vi "GTcode_v6_simulISS_MAP.vi"() -> ()   [LabVIEW 2016]
uses:
  <vilib>/Utility/config.llb/Write Key (String).vi
  <vilib>/Utility/config.llb/Write Key (U32).vi
  <vilib>/Utility/config.llb/Write Key (Double).vi
  <vilib>/Utility/config.llb/Write Key (I32).vi
  <vilib>/Utility/config.llb/Read Key (U32).vi
  <vilib>/Utility/config.llb/Read Key (I32).vi
  flex05-4chPascal.dll
  <vilib>/Utility/config.llb/NI_LVConfig.lvlib
  flex05oem8chauto100nsPASCAL_win7.dll
  <vilib>/Analysis/NI_AALBase.lvlib
panel:
  in  "Tab Control":T1(tab)=enum."Real Time Fitting Parameters"
  out "COV":dbl
  out "mean":dbl format="%0.2f"
  in  "Fixed Time":bool
  in  "Detector Used":T2(ring)=enum."Det 2"
  in  "Real Time Fitting?":bool
  out "g2":cluster{"Delay Time":sgl[], sgl[]}[](graph) caption="Normalized Correlation Function"
  out "Tau":cluster{"tmp":dbl, dbl}(graph) caption="Relative Changes of Flow"
  in  "QUIT":bool
  in  "Clear plots":bool
  in  "Baseline":bool
  in  "MARK\nMark":bool
  in  "Stop":bool
  in  "Sequence Scan":bool
  out "Mark #":u32
  out "Trial #":u32
  out "Frame #":u32
  out "Det 8":sgl format="%.3f"
  out "Det 7":sgl format="%.3f"
  out "Det 6":sgl format="%.3f"
  out "Det 5":sgl format="%.3f"
  out "Det 4":sgl format="%.3f"
  out "Det 3":sgl format="%.3f"
  out "Det 2":sgl format="%.3f"
  out "Det 1":sgl format="%.3f"
  out "Computer Time":string="2010-1-12 23:16:10"
  in  "D1":bool
  in  "D2":bool
  in  "D3":bool
  in  "D4":bool
  in  "D5":bool
  in  "D6":bool
  in  "D7":bool
  in  "D8":bool
  out "Tau 2":T3(graph)={1.6593152555505744e-08, 3.9427894777554196e-08, 4.065716407938411e-08, 1.5135790977358522e-08, 2.4870420100428357e-08, 7.094765128107397e-08, 0.0, 4.1348620928852906e-07, 1.5886917674344795e-08, 4.0280526032721455e-08, -1.0, -1.0} caption="Blood Flow Index (cm2/s)"
  in  "Fixed # of Frames":u32=5
  out "Status":string="Quit"
  in  "Optical Switch OPEN":bool
  in  "Delay between frames(ms)":u32=500
  out "Time Left (ms)":sgl format="%.3f"
  in  "Integration Time (ms)":sgl=1000.0 min=1 max=13000 step=1
  in  "File Name:":string="test0"
  in  "Data Save Directory:":path=path "C:/data"
  in  "ISS Lasers ON":bool
  in  "Test":bool
  in  "Lines":tag="Dev1/port1/line0:1, Dev1/port1/line3:7"
  in  "Delaytime(ms)":u32=200
  in  "Initialize Correlator":bool
  in  "Detector Select":enum32{"4 Detectors", "8 Detectors"}(radio)=enum."8 Detectors"
  in  "Update Time (ms)\nDO NOT CHANGE!":u32=105 min=1 max=999 step=1
  in  "Laser Input Name":refnum<visa-resource-name>="COM7"
  out "Flow in each detector":dbl[](array[numeric])=[-1.0, -1.0, -1.0, -1.0, -1.0, -1.0, -1.0, -1.0, -1.0, -1.0, -1.0, -1.0]
  in  "Visible Averages":bool[](array[boolean])=[FALSE, FALSE, FALSE, FALSE]
  in  "Avg":bool[][](array[boolean])=[[FALSE, FALSE, FALSE, FALSE, FALSE, FALSE, FALSE, FALSE], [FALSE, FALSE, FALSE, FALSE, FALSE, FALSE, FALSE, FALSE], [FALSE, FALSE, FALSE, FALSE, FALSE, FALSE, FALSE, FALSE], [FALSE, FALSE, FALSE, FALSE, FALSE, FALSE, FALSE, FALSE]]
  in  "rho":dbl[](array[numeric])=[2.5, 2.5, 2.5, 2.5, 2.5, 2.5, 2.5, 2.5, -1.0, -1.0, -1.0, -1.0]
  in  "Other Settings":u32[](array[numeric])=[1, 120, 0, 1] caption="Flow in each detector"
  in  "Initial Guess":dbl[](array[numeric])=[1e-08, 0.5, 0.05, 10.0] caption="Flow in each detector"
  in  "Number Samples":dbl=50.0
  out "NIBP Data (*scaled by 98 to convert from V to mmHg)":dynamicdata(graph)
  in  "Record MAP data?":bool=TRUE
  in  "Sampling Rate (Hz)":dbl=100.0
  in  "ExternalADC":tag="Dev2"
  out "4CH?":bool
  out "Detector#":u32=1
  out "Source#":u32=1
  # "kHz"
  # "kHz"
  # "Don't Change these Parameters unless you know clearly what you are doing"
  # "ISS Triggers Setup"
  # "Channel Parameters"
  # "Step1"
  # "Line"
  # "0"
  # "1"
  # "3"
  # "4"
  # "5"
  # "6"
  # "7"
  # "*The number of lines in the list must\nmatch the number of elements in\nthe array."
  # "Step2"
  # "Line"
  # "0"
  # "1"
  # "3"
  # "4"
  # "5"
  # "6"
  # "7"
  # "Step3"
  # "Line"
  # "0"
  # "1"
  # "3"
  # "4"
  # "5"
  # "6"
  # "7"
  # "Line    Signal\n\n0           ISS Trigger (0: OFF, 1: ON)\n1           Flow Laser 1 ON/OFF (0:OFF, 1:ON)\n2           ISS Data Acquisition (0: DONE, 1: NO)\n3           ISS Laser ON/OFF (0: ON, 1: OFF)\n4           Trigger for Marks  (0: OFF, 1: ON)\n5           Flow Laser 2 ON/OFF (0:OFF, 1:ON)\n6           Reserved\n7           Reserved"
  # "Wait ISS Data Acuisition DONE Signal"
  # "Step4"
  # "Step5"
  # "Line"
  # "0"
  # "1"
  # "3"
  # "4"
  # "5"
  # "6"
  # "7"
  # "Flow Lasers Setup"
  # "FROM FRONT PANEL"
  # "Line"
  # "0"
  # "1"
  # "3"
  # "4"
  # "5"
  # "6"
  # "7"
  # "Line"
  # "0"
  # "1"
  # "3"
  # "4"
  # "5"
  # "6"
  # "7"
  # "Det 1"
  # "Det 2"
  # "Det 3"
  # "Det 4"
  # "Det 5"
  # "Det 6"
  # "Det 7"
  # "Det 8"
  # "Avg 1"
  # "Avg 2"
  # "Avg 3"
  # "Avg 4"
  # "Db"
  # "Beta"
  # "Mua"
  # "MuS'"
  # "1"
  # "2"
  # "3"
  # "4"
  # "5"
  # "6"
  # "7"
  # "8"
  # "Avg 1"
  # "Starting Pt"
  # "End Pt"
  # "Approximate"
  # "Variables"
  # "Avg 2"
  # "Avg 3"
  # "Avg 4"
  # "Source Detector  Separations"
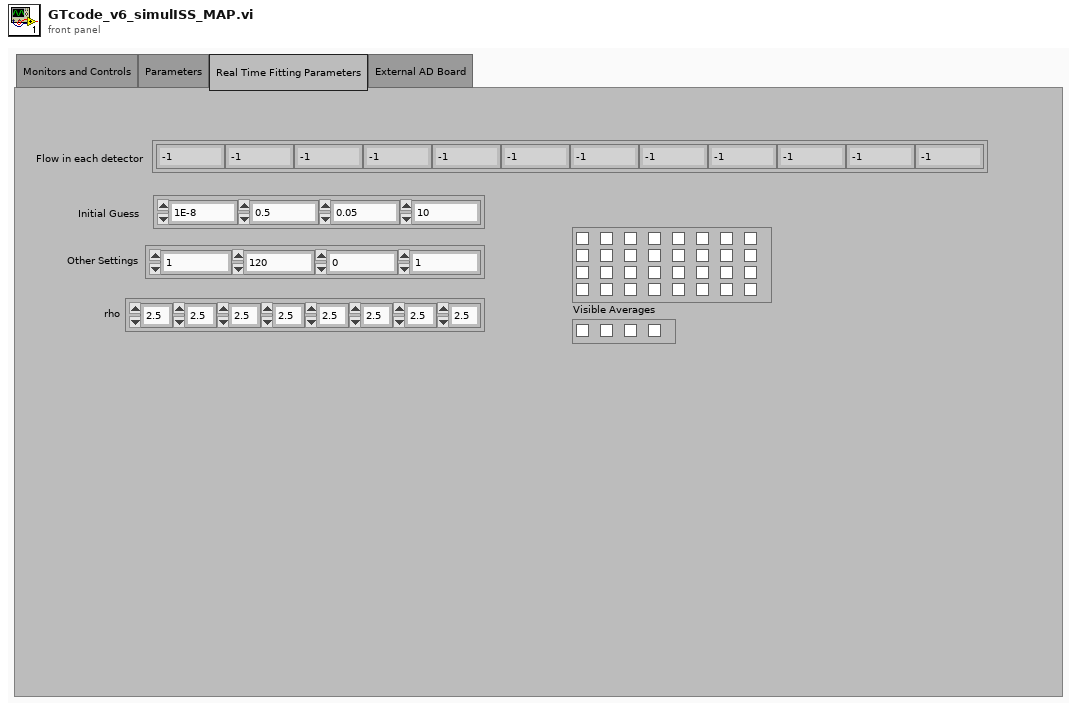
[diagram p1: front panel]
types:
  T1 = enum32{"Monitors and Controls", "Parameters", "Real Time Fitting Parameters", "External AD Board"}
  T2 = enum16{"Det 1", "Det 2", "Det 3", "Det 4", "Det 5", "Det 6", "Det 7", "Det 8"}
  T3 = cluster{dbl, dbl, dbl, dbl, dbl, dbl, dbl, dbl, dbl, dbl, dbl, dbl}
  T4 = enum8{"Enabled", "Disabled", "Disabled and Grayed Out"}
  T5 = cluster{dbl, dbl, dbl, dbl, dbl, dbl, dbl, dbl, dbl, dbl, dbl, dbl}[]
  T6 = typedef "NI_LVConfig.lvlib/Config Data RefNum.ctl" = refnum<k1>
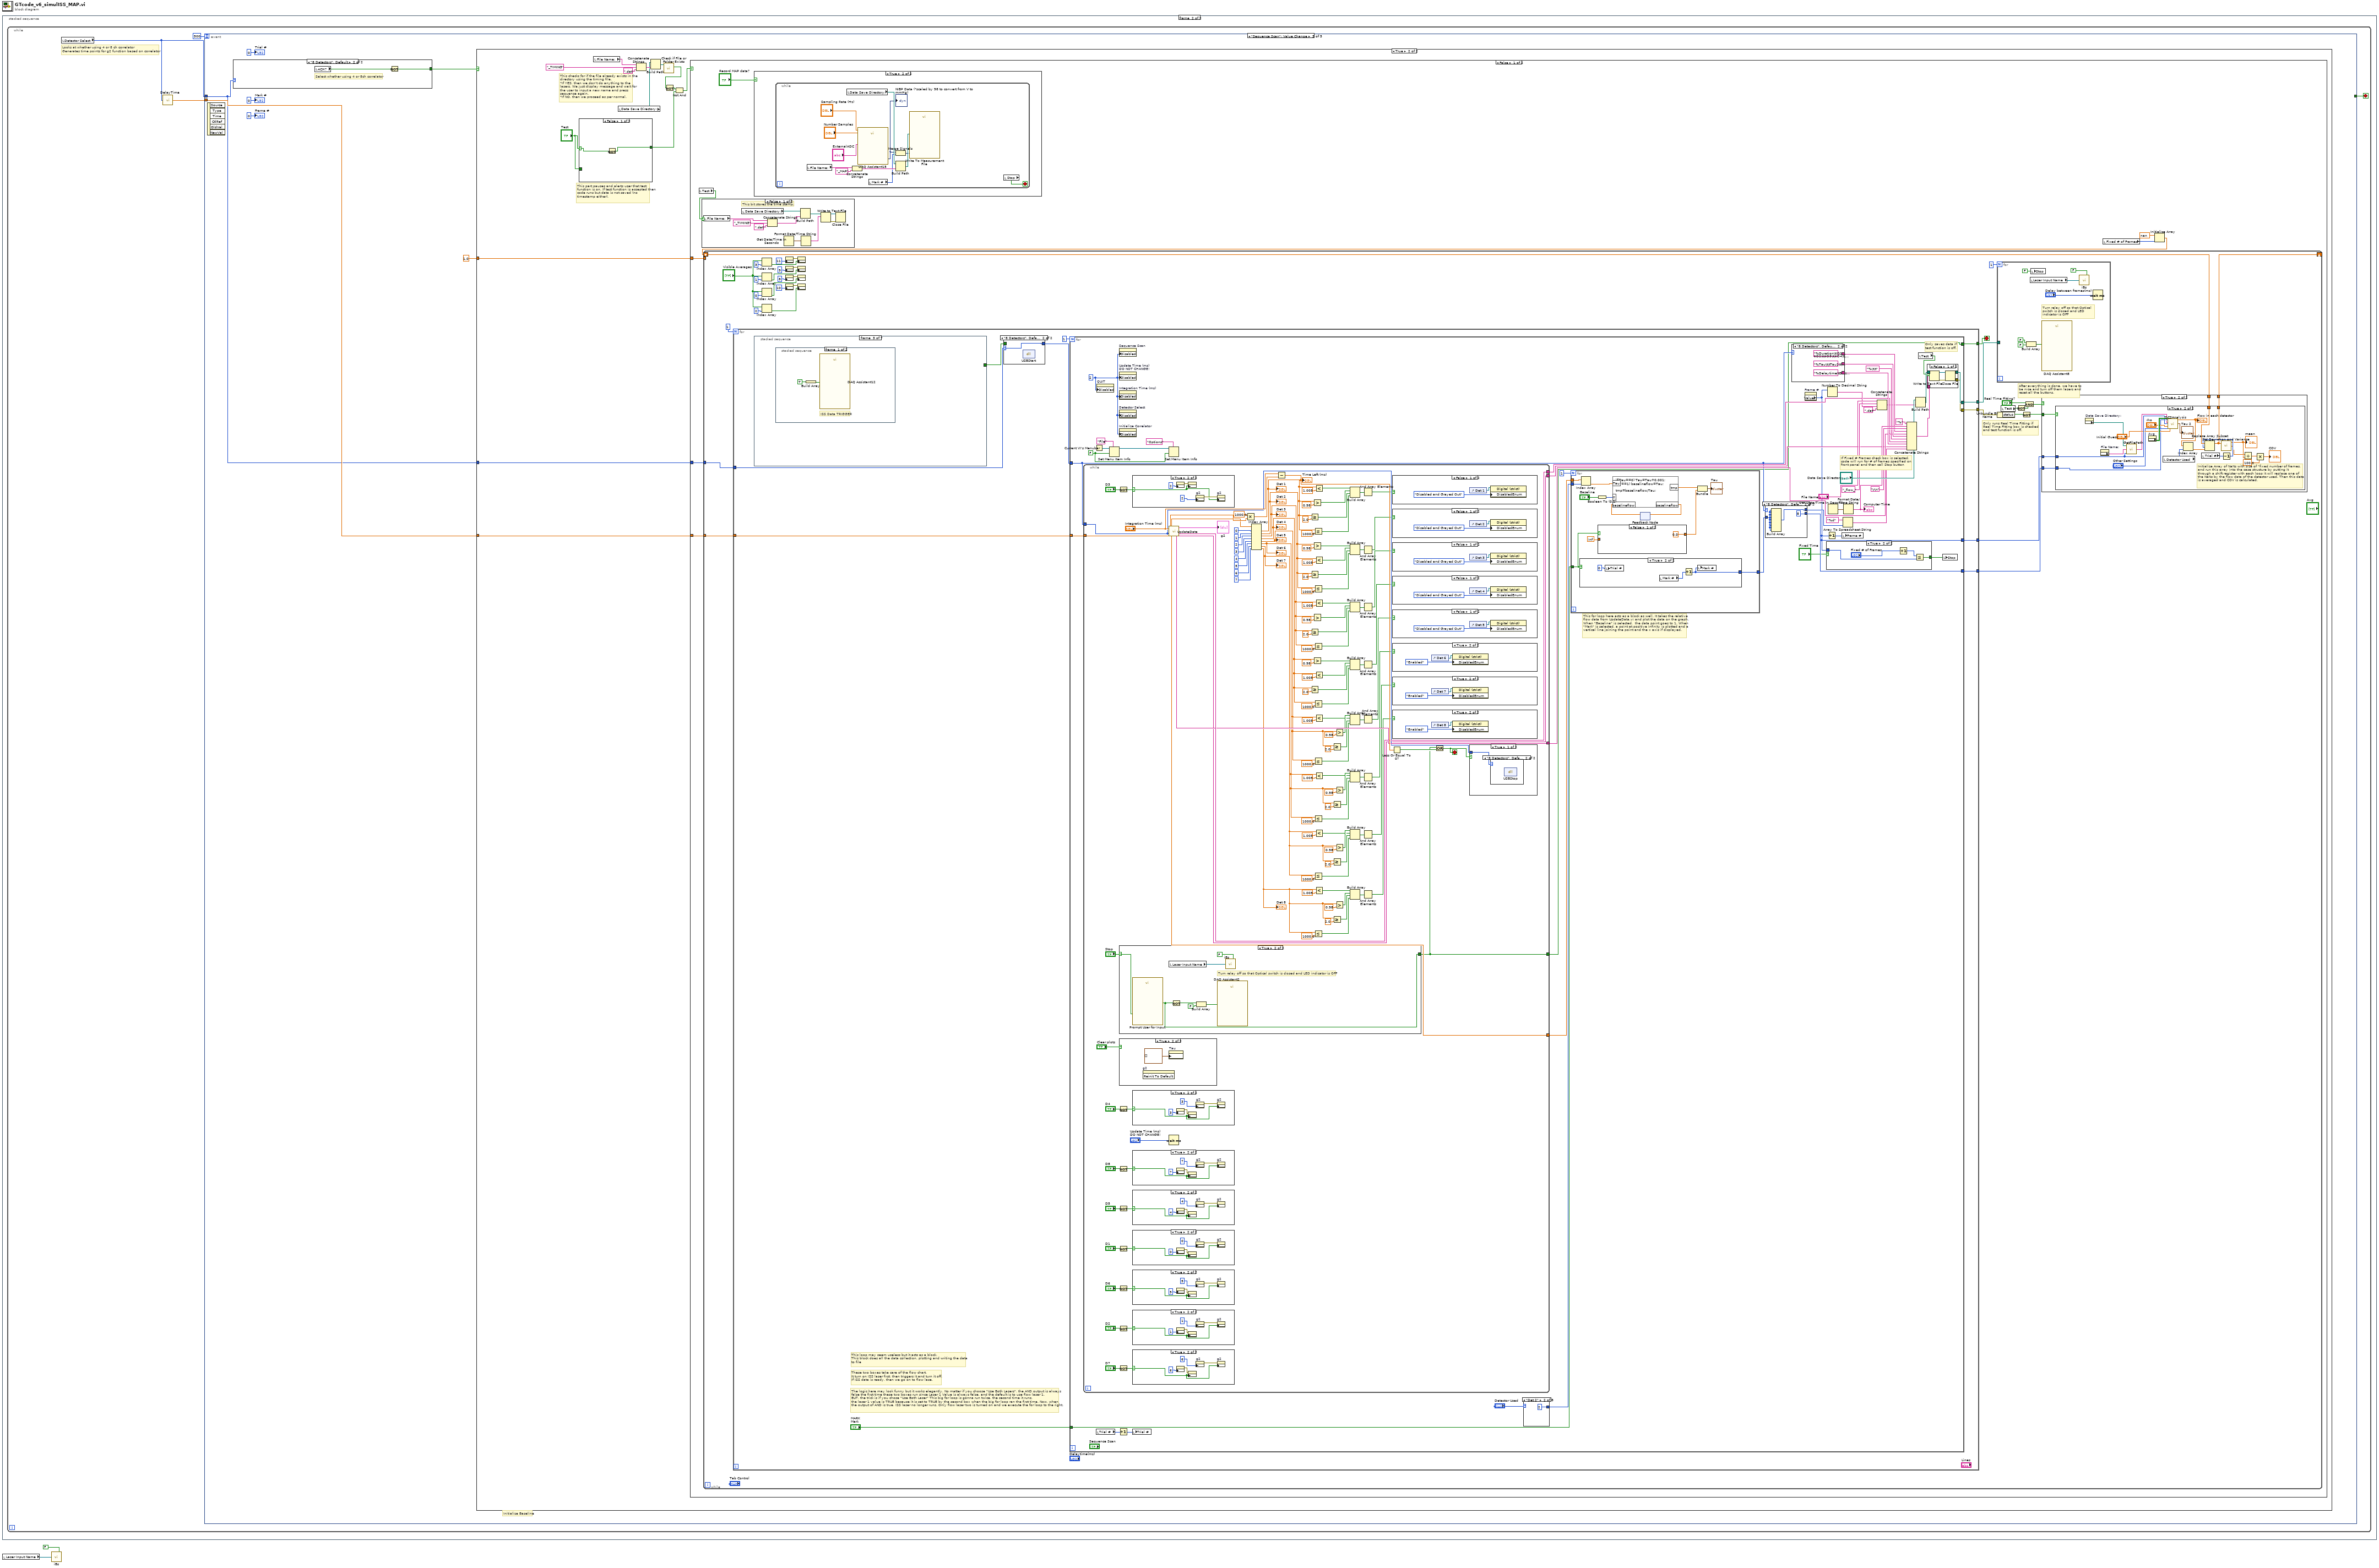
[diagram p0: block diagram]
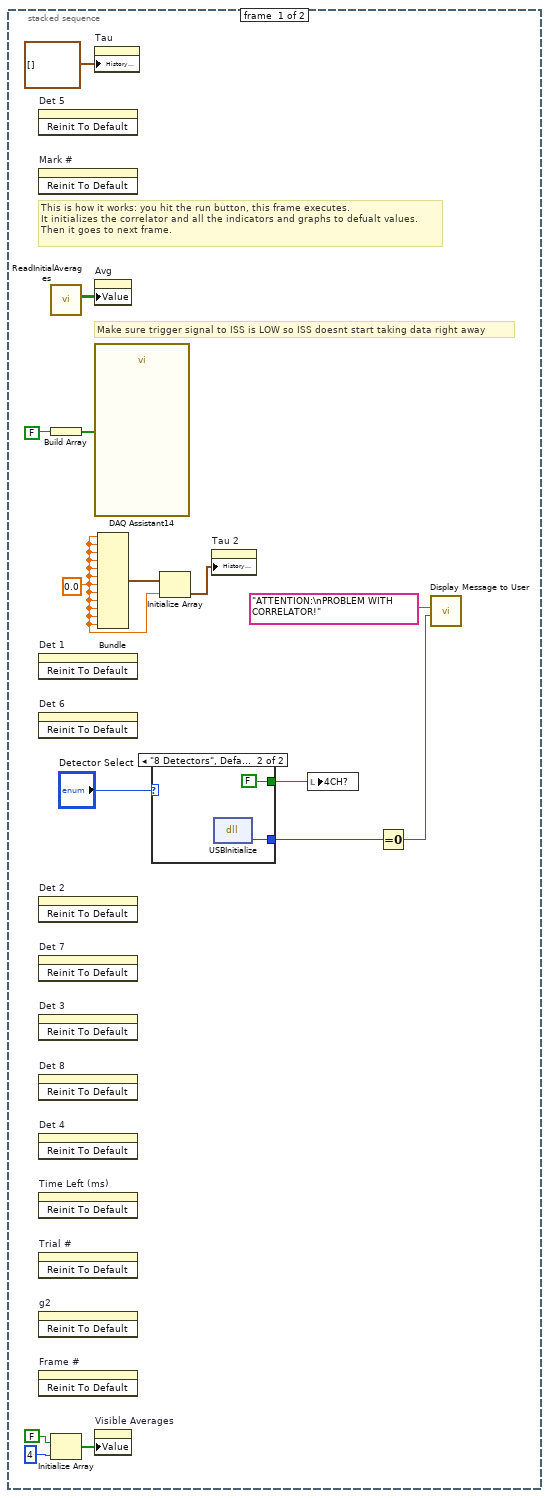
[diagram p2: hidden frame]
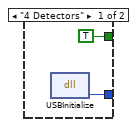
[diagram p3: hidden frame]
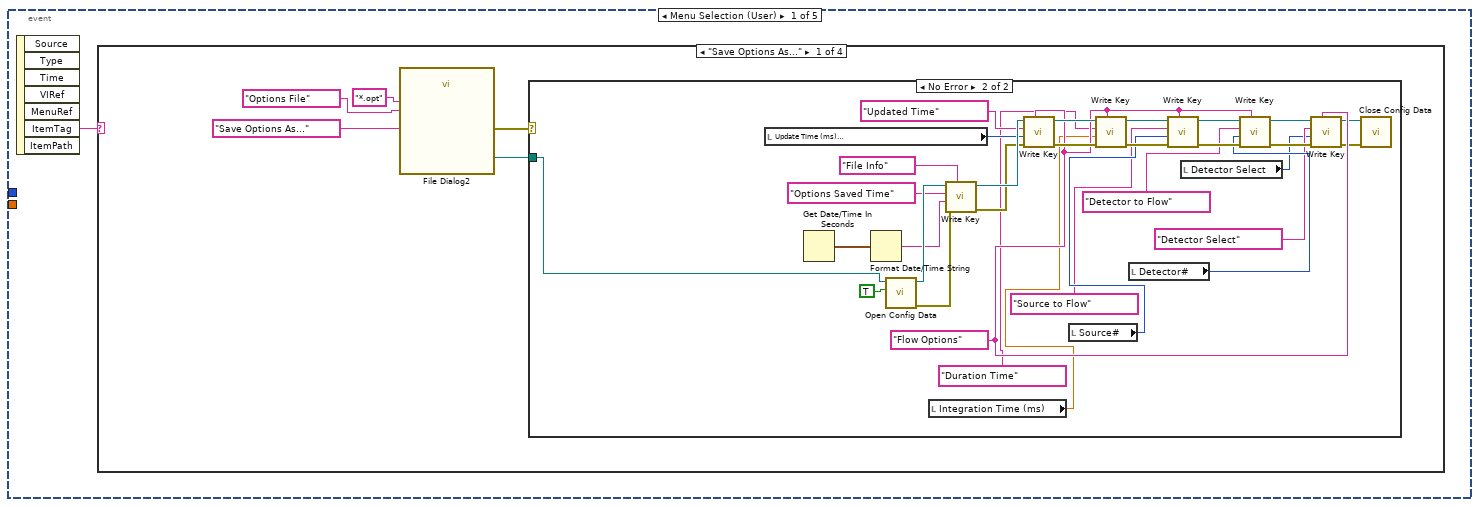
[diagram p4: hidden frame]
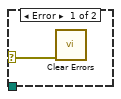
[diagram p5: hidden frame]
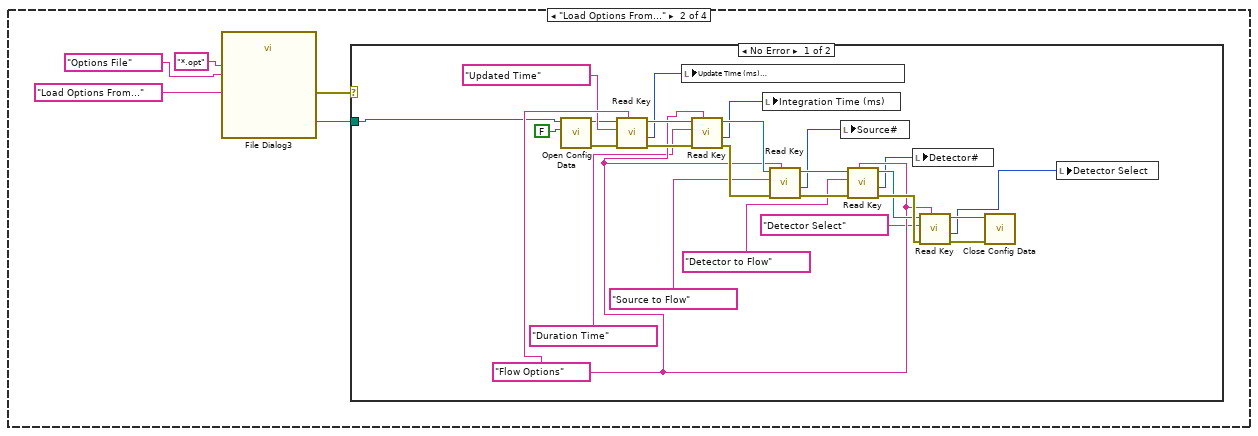
[diagram p6: hidden frame]
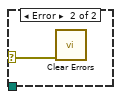
[diagram p7: hidden frame]
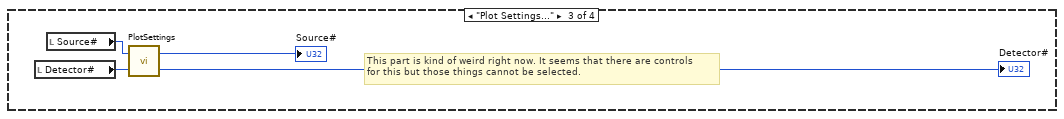
[diagram p8: hidden frame]
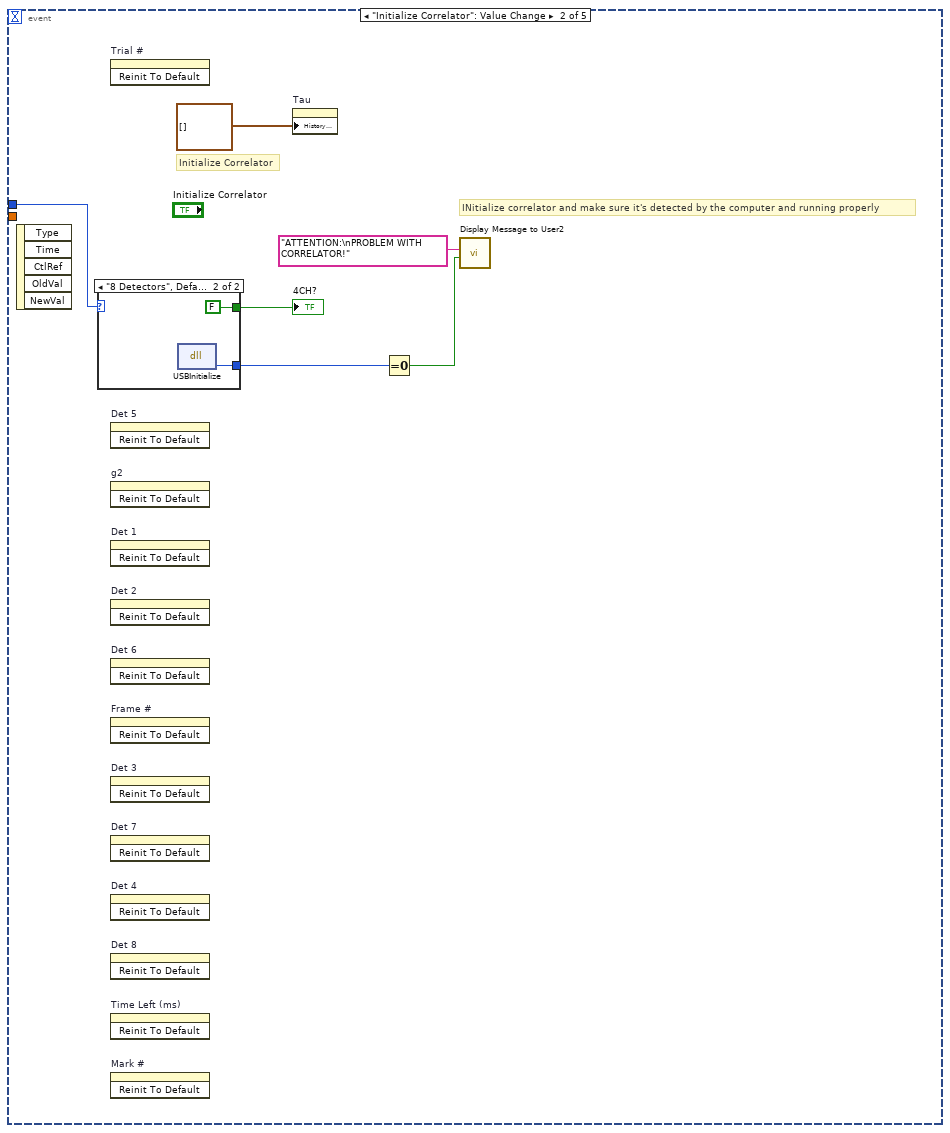
[diagram p10: hidden frame]
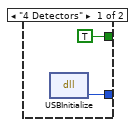
[diagram p11: hidden frame]
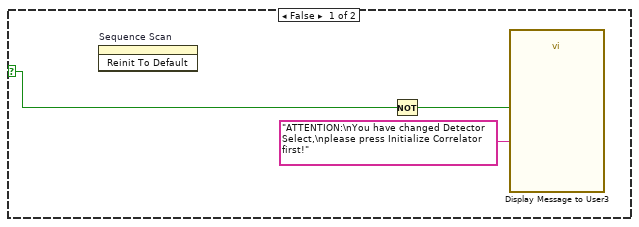
[diagram p12: hidden frame]
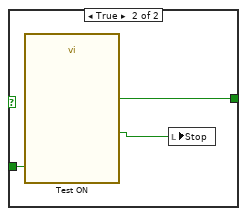
[diagram p13: hidden frame]
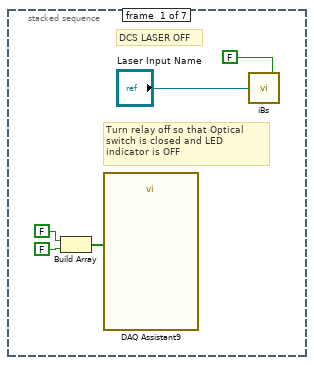
[diagram p18: hidden frame]
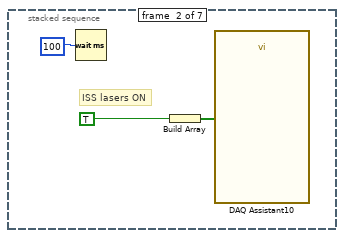
[diagram p19: hidden frame]
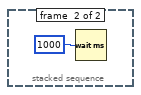
[diagram p20: hidden frame]
diagram:
  n1 = stacked-sequence {
    frame #0 {
      w7 = 0.0
      # "Make sure trigger signal to ISS is LOW so ISS doesnt start taking data right away"
      # "This is how it works: you hit the run button, this frame executes.\nIt initializes the correlator and all the indicators and graphs to defualt values.\nThen it goes to next frame."
      n2 = invoke on="Det 5" class="DigNum (strict)" method="Reinit To Default"() -> ()  [unwired: 3 in, 3 out]
      n3 = invoke on="Mark #" class="DigNum (strict)" method="Reinit To Default"() -> ()  [unwired: 3 in, 3 out]
      n4 = invoke on="Det 1" class="DigNum (strict)" method="Reinit To Default"() -> ()  [unwired: 3 in, 3 out]
      n5 = invoke on="Det 6" class="DigNum (strict)" method="Reinit To Default"() -> ()  [unwired: 3 in, 3 out]
      n6 = invoke on="Det 2" class="DigNum (strict)" method="Reinit To Default"() -> ()  [unwired: 3 in, 3 out]
      n7 = invoke on="Det 7" class="DigNum (strict)" method="Reinit To Default"() -> ()  [unwired: 3 in, 3 out]
      n8 = invoke on="Det 3" class="DigNum (strict)" method="Reinit To Default"() -> ()  [unwired: 3 in, 3 out]
      n9 = invoke on="Det 8" class="DigNum (strict)" method="Reinit To Default"() -> ()  [unwired: 3 in, 3 out]
      n10 = invoke on="Det 4" class="DigNum (strict)" method="Reinit To Default"() -> ()  [unwired: 3 in, 3 out]
      n11 = invoke on="Time Left (ms)" class="DigNum (strict)" method="Reinit To Default"() -> ()  [unwired: 3 in, 3 out]
      n12 = invoke on="Trial #" class="DigNum (strict)" method="Reinit To Default"() -> ()  [unwired: 3 in, 3 out]
      n13 = invoke on="g2" class="XYGraph (strict)" method="Reinit To Default"() -> ()  [unwired: 3 in, 3 out]
      n14 = invoke on="Frame #" class="DigNum (strict)" method="Reinit To Default"() -> ()  [unwired: 3 in, 3 out]
      n15 = call "ReadInitialAverages.vi"() -> ("avgOut"=w6:bool[][])  [unwired: 11 in]
      n16 = Build Array(FALSE) -> (w3:bool[])
      n17 = Initialize Array(FALSE, 4) -> (w5:bool[])
      n18 = property on="Tau" class="WFChart (strict)"("History Data"=cluster{"tmp":dbl, dbl}[] []) -> ()  [unwired: 2 in, 2 out]
      n19 = property on="Avg" class="Arr (strict)"("Value"=w6) -> ()  [unwired: 2 in, 2 out]
      n20 = call "DAQ Assistant14"("data"=w3) -> ()  [unwired: 17 in, 2 out]
      n21 = property on="Visible Averages" class="Arr (strict)"("Value"=w5) -> ()  [unwired: 2 in, 2 out]
      n22 = Bundle(w7, w7, w7, w7, w7, w7, w7, w7, w7, w7, w7, w7) -> (w9:T3)  [unwired: 1 in]
      n23 = case shown="\"8 Detectors\", Default" "Detector Select" {
        tunnel: [w19 w21] -> w17
        tunnel: [TRUE FALSE] -> w15
        frame "4 Detectors" {
          n24 = dll-call lib="C:/Users/BUCKLEY-ADMIN/Desktop/DCScode_simulISS_MAP/flex05-4chPascal.dll" fn="USBInitialize" label="InitCH4"() -> ("return type"=w19:u8)  [unwired: 3 in, 2 out]
        }
        frame "8 Detectors", Default {
          n25 = dll-call lib="C:/Users/BUCKLEY-ADMIN/Desktop/DCScode_simulISS_MAP/flex05oem8chauto100nsPASCAL_win7.dll" fn="USBInitialize" label="InitCH8"() -> ("return type"=w21:u8)  [unwired: 3 in, 2 out]
        }
      }
      n26 = Initialize Array(w9, w7) -> (w8:T5)
      n27 = property on="Tau 2" class="WFChart (strict)"("History Data"=w8) -> ()  [unwired: 2 in, 2 out]
      n28 = local write "4CH?"(w15) -> ()
      n29 = Equal To 0?(x=w17) -> (x = 0?=w16:bool)
      n30 = call "Display Message to User"("Enable"=w16, "Message"="ATTENTION:\nPROBLEM WITH CORRELATOR!") -> ()  [unwired: 8 in, 2 out]
    }
    frame #1 {
      n31 = while {
        stop <- w25 stop-if-true
        # "Looks at whether using 4 or 8 ch correlator\nGenerates time points for g2 function based on correlator"
        n32 = local read "Detector Select"() -> (w22:enum32{"4 Detectors", "8 Detectors"})
        n33 = call "DelayTime.vi"("Detector Select"=w22) -> ("Delaytime"=w23:sgl[])
        n34 = event shown="[2] \"Sequence Scan\": Value Change" {
          selector: _ -> [_ _ _ _ _]
          dyn-events: _ -> [_ _ _ _ _]
          timeout: 500 -> [_ _ _ _ _]
          tunnel: w23 -> [_ _ w115 _ _]
          tunnel: [_ _ _ "QUIT" _] -> w25
          tunnel: w22 -> [_ w102 w111 w617 _]
          event Menu Selection (User) {
            n35 = event-data() -> ("ItemTag"=w26:string)  [unwired: 1 in, 6 out]
            n36 = case shown="\"Save Options As...\"" w26 {
              frame "Save Options As..." {
                n37 = call "File Dialog2"("prompt"="Save Options As...", "pattern (all files)"="*.opt", "pattern label"="Options File") -> ("selected path"=w28:path, "error out"=w27:errorcluster)  [unwired: 9 in, 2 out]
                n38 = case shown="No Error" w27 {
                  selector: w27 -> [w32 _]
                  tunnel: w28 -> [_ w63]
                  frame Error {
                    n39 = call <vilib>:"Clear Errors.vi"("error in (no error)"=w32) -> ()  [unwired: 5 in, 2 out]
                  }
                  frame No Error {
                    w50 = "Flow Options"
                    n40 = local read "Update Time (ms)\nDO NOT CHANGE!"() -> (w43:u32)
                    n41 = Get Date/Time In Seconds() -> (seconds since 1Jan1904=w49:timestamp)
                    n42 = Format Date/Time String(seconds (now)=w49) -> (date/time string=w45:string)  [unwired: 2 in]
                    n43 = call <vilib>:"Open Config Data.vi"("create file if necessary (T)"=TRUE, "configuration file path"=w63) -> ("error out"=w61:errorcluster, "refnum"=w60:T6)  [unwired: 7 in, 1 out]
                    n44 = local read "Integration Time (ms)"() -> (w41:sgl)
                    n45 = call-poly <vilib>:"Write Key.vi"("section"="File Info", "error in (no error)"=w61, "value"=w45, "key"="Options Saved Time", "refnum"=w60) -> ("error out"=w47:errorcluster, "refnum out"=w48:T6)  [unwired: 4 in, 1 out]
                    n46 = call-poly <vilib>:"Write Key.vi"("section"=w50, "error in (no error)"=w47, "value"=w43, "key"="Updated Time", "refnum"=w48) -> ("error out"=w59:errorcluster, "refnum out"=w58:T6)  [unwired: 4 in, 1 out]
                    n47 = local read "Source#"() -> (w40:u32)
                    n48 = call-poly <vilib>:"Write Key.vi"("section"=w50, "error in (no error)"=w59, "value"=w41, "key"="Duration Time", "refnum"=w58) -> ("error out"=w54:errorcluster, "refnum out"=w55:T6)  [unwired: 4 in, 1 out]
                    n49 = local read "Detector#"() -> (w37:u32)
                    n50 = call-poly <vilib>:"Write Key.vi"("section"=w50, "error in (no error)"=w54, "value"=w40, "key"="Source to Flow", "refnum"=w55) -> ("error out"=w56:errorcluster, "refnum out"=w57:T6)  [unwired: 4 in, 1 out]
                    n51 = local read "Detector Select"() -> (w35:enum32{"4 Detectors", "8 Detectors"})
                    n52 = call-poly <vilib>:"Write Key.vi"("section"=w50, "error in (no error)"=w56, "value"=w37, "key"="Detector to Flow", "refnum"=w57) -> ("error out"=w53:errorcluster, "refnum out"=w52:T6)  [unwired: 4 in, 1 out]
                    n53 = call-poly <vilib>:"Write Key.vi"("section"=w50, "error in (no error)"=w53, "value"=w35, "key"="Detector Select", "refnum"=w52) -> ("error out"=w33:errorcluster, "refnum out"=w34:T6)  [unwired: 4 in, 1 out]
                    n54 = call <vilib>:"Close Config Data.vi"("error in (no error)"=w33, "refnum"=w34) -> ()  [unwired: 8 in, 2 out]
                  }
                }
              }
              frame "Load Options From..." {
                n55 = call "File Dialog3"("prompt"="Load Options From...", "pattern (all files)"="*.opt", "pattern label"="Options File") -> ("selected path"=w65:path, "error out"=w64:errorcluster)  [unwired: 9 in, 2 out]
                n56 = case shown="No Error" w64 {
                  selector: w64 -> [_ w94]
                  tunnel: w65 -> [w69 _]
                  frame No Error {
                    w84 = "Flow Options"
                    n57 = call <vilib>:"Open Config Data.vi"("create file if necessary (T)"=FALSE, "configuration file path"=w69) -> ("error out"=w76:errorcluster, "refnum"=w75:T6)  [unwired: 7 in, 1 out]
                    n58 = call-poly <vilib>:"Read Key.vi"("section"=w84, "error in (no error)"=w76, "key"="Updated Time", "refnum"=w75) -> ("error out"=w92:errorcluster, "value"=w74:u32, "refnum out"=w91:T6)  [unwired: 4 in, 1 out]
                    n59 = local write "Update Time (ms)\nDO NOT CHANGE!"(w74) -> ()
                    n60 = call-poly <vilib>:"Read Key.vi"("section"=w84, "error in (no error)"=w92, "key"="Duration Time", "refnum"=w91) -> ("error out"=w87:errorcluster, "value"=w73:i32, "refnum out"=w88:T6)  [unwired: 4 in, 1 out]
                    n61 = local write "Integration Time (ms)"(w73) -> ()
                    n62 = call-poly <vilib>:"Read Key.vi"("section"=w84, "error in (no error)"=w87, "key"="Source to Flow", "refnum"=w88) -> ("error out"=w89:errorcluster, "value"=w70:u32, "refnum out"=w90:T6)  [unwired: 4 in, 1 out]
                    n63 = local write "Source#"(w70) -> ()
                    n64 = call-poly <vilib>:"Read Key.vi"("section"=w84, "error in (no error)"=w89, "key"="Detector to Flow", "refnum"=w90) -> ("error out"=w86:errorcluster, "value"=w71:u32, "refnum out"=w85:T6)  [unwired: 4 in, 1 out]
                    n65 = local write "Detector#"(w71) -> ()
                    n66 = call-poly <vilib>:"Read Key.vi"("section"=w84, "error in (no error)"=w86, "key"="Detector Select", "refnum"=w85) -> ("error out"=w77:errorcluster, "value"=w72:u32, "refnum out"=w78:T6)  [unwired: 4 in, 1 out]
                    n67 = call <vilib>:"Close Config Data.vi"("error in (no error)"=w77, "refnum"=w78) -> ()  [unwired: 8 in, 2 out]
                    n68 = local write "Detector Select"(w72) -> ()
                  }
                  frame Error {
                    n69 = call <vilib>:"Clear Errors.vi"("error in (no error)"=w94) -> ()  [unwired: 5 in, 2 out]
                  }
                }
              }
              frame "Plot Settings..." {
                # "This part is kind of weird right now. It seems that there are controls\nfor this but those things cannot be selected."
                n70 = local read "Detector#"() -> (w96:u32)
                n71 = local read "Source#"() -> (w97:u32)
                n72 = call "PlotSettings.vi"("Detectorin"=w96, "Sourcein"=w97) -> ("Detector#"=→"Detector#":u32, "Source#"=→"Source#":u32)
              }
              frame Default {
              }
            }
          }
          event "Initialize Correlator": Value Change {
            # "INitialize correlator and make sure it's detected by the computer and running properly"
            # "Initialize Correlator"
            n73 = event-data() -> ()  [unwired: 1 in, 5 out]
            n74 = case shown="\"8 Detectors\", Default" w102 {
              tunnel: [w106 w108] -> w104
              tunnel: [TRUE FALSE] -> w101
              frame "4 Detectors" {
                n75 = dll-call lib="C:/Users/BUCKLEY-ADMIN/Desktop/DCScode_simulISS_MAP/flex05-4chPascal.dll" fn="USBInitialize" label="InitCH4"() -> ("return type"=w106:u8)  [unwired: 3 in, 2 out]
              }
              frame "8 Detectors", Default {
                n76 = dll-call lib="C:/Users/BUCKLEY-ADMIN/Desktop/DCScode_simulISS_MAP/flex05oem8chauto100nsPASCAL_win7.dll" fn="USBInitialize" label="InitCH8"() -> ("return type"=w108:u8)  [unwired: 3 in, 2 out]
              }
            }
            "4CH?" <- w101
            n77 = invoke on="Trial #" class="DigNum (strict)" method="Reinit To Default"() -> ()  [unwired: 3 in, 3 out]
            n78 = invoke on="Det 5" class="DigNum (strict)" method="Reinit To Default"() -> ()  [unwired: 3 in, 3 out]
            n79 = invoke on="g2" class="XYGraph (strict)" method="Reinit To Default"() -> ()  [unwired: 3 in, 3 out]
            n80 = invoke on="Det 1" class="DigNum (strict)" method="Reinit To Default"() -> ()  [unwired: 3 in, 3 out]
            n81 = invoke on="Det 2" class="DigNum (strict)" method="Reinit To Default"() -> ()  [unwired: 3 in, 3 out]
            n82 = invoke on="Det 6" class="DigNum (strict)" method="Reinit To Default"() -> ()  [unwired: 3 in, 3 out]
            n83 = invoke on="Frame #" class="DigNum (strict)" method="Reinit To Default"() -> ()  [unwired: 3 in, 3 out]
            n84 = invoke on="Det 3" class="DigNum (strict)" method="Reinit To Default"() -> ()  [unwired: 3 in, 3 out]
            n85 = invoke on="Det 7" class="DigNum (strict)" method="Reinit To Default"() -> ()  [unwired: 3 in, 3 out]
            n86 = invoke on="Det 4" class="DigNum (strict)" method="Reinit To Default"() -> ()  [unwired: 3 in, 3 out]
            n87 = invoke on="Det 8" class="DigNum (strict)" method="Reinit To Default"() -> ()  [unwired: 3 in, 3 out]
            n88 = invoke on="Time Left (ms)" class="DigNum (strict)" method="Reinit To Default"() -> ()  [unwired: 3 in, 3 out]
            n89 = invoke on="Mark #" class="DigNum (strict)" method="Reinit To Default"() -> ()  [unwired: 3 in, 3 out]
            n90 = property on="Tau" class="WFChart (strict)"("History Data"=cluster{"tmp":dbl, dbl}[] []) -> ()  [unwired: 2 in, 2 out]
            n91 = Equal To 0?(x=w104) -> (x = 0?=w103:bool)
            n92 = call "Display Message to User2"("Enable"=w103, "Message"="ATTENTION:\nPROBLEM WITH CORRELATOR!") -> ()  [unwired: 8 in, 2 out]
          }
          event "Sequence Scan": Value Change {
            # "Initialize Baseline"
            n93 = event-data() -> ()  [unwired: 1 in, 6 out]
            n94 = case shown="\"8 Detectors\", Default" w111 {
              tunnel: [w612 w613] -> w110
              frame "4 Detectors" {
                n95 = local read "4CH?"() -> (w612:bool)
              }
              frame "8 Detectors", Default {
                # "Select whether using 4 or 8ch correlator"
                n96 = local read "4CH?"() -> (w614:bool)
                n97 = Not(x=w614) -> (.not. x?=w613:bool)
              }
            }
            n98 = case shown="True" w110 {
              selector: w110 -> [w117 _]
              tunnel: w115 -> [_ w131]
              tunnel: w111 -> [_ w132]
              tunnel: sgl 1.0 -> [_ w130]
              frame False {
                n99 = invoke on="Sequence Scan" class="Bool" method="Reinit To Default"() -> ()  [unwired: 3 in, 3 out]
                n100 = Not(x=w117) -> (.not. x?=w116:bool)
                n101 = call "Display Message to User3"("Enable"=w116, "Message"="ATTENTION:\nYou have changed Detector Select,\nplease press Initialize Correlator first!") -> ()  [unwired: 8 in, 2 out]
              }
              frame True {
                # "This part pauses and alerts user that test function is on. If test function is accepted then code runs but data is not saved (no timestamp either)."
                # "This checks for if the file already exists in the\ndirectory using the timing file. \n*If YES, then we don't do anything to the lasers. We just display message and wait for the user to input a new name and press sequence again.\n*If NO, then we proceed as per normal."
                n102 = case shown="False" "Test" {
                  selector: "Test" -> [w134 _]
                  tunnel: "Test" -> [_ w136]
                  tunnel: [w133 w135] -> w120
                  frame False {
                    n103 = Not(x=w134) -> (.not. x?=w133:bool)
                  }
                  frame True {
                    n104 = call "Test ON"("Enable"=w136) -> ("No - STOP"=w137:bool, "OK"=w135:bool)  [unwired: 15 in, 2 out]
                    n105 = local write "Stop"(w137) -> ()
                  }
                }
                n106 = local read "File Name:"() -> (w126:string)
                n107 = local read "Data Save Directory:"() -> (w125:path)
                n108 = Concatenate Strings(w126, "_TIMING", ".dat") -> (w128:string)
                n109 = Build Path(base path=w125, name or relative path=w128) -> (appended path=w124:path)
                n110 = call <vilib>:"Check if File or Folder Exists.vi"("path"=w124) -> ("file or folder exists?"=w122:bool)  [unwired: 8 in, 2 out]
                n111 = Not(x=w122) -> (.not. x?=w123:bool)
                n112 = Not And(1:w120, 2:w123) -> (0:w121:bool)
                n113 = case shown="False" w121 {
                  tunnel: w132 -> [w145 _]
                  tunnel: w131 -> [w144 _]
                  tunnel: w130 -> [w143 _]
                  frame False {
                    n114 = local read "Test"() -> (w141:bool)
                    n115 = case shown="False" w141 {
                      frame False {
                        # "This bit stores the time stamp."
                        n116 = local read "File Name:"() -> (w146:string)
                        n117 = local read "Data Save Directory:"() -> (w147:path)
                        n118 = Concatenate Strings(w146, "_TIMING", ".dat") -> (w151:string)
                        n119 = Get Date/Time In Seconds() -> (seconds since 1Jan1904=w148:timestamp)
                        n120 = Build Path(base path=w147, name or relative path=w151) -> (appended path=w150:path)
                        n121 = Format Date/Time String(seconds (now)=w148) -> (date/time string=w154:string)  [unwired: 2 in]
                        n122 = Write to Text File(file (use dialog)=w150, text=w154) -> (refnum out=w153:refnum<file>, error out=w152:errorcluster)  [unwired: 2 in, 1 out]
                        n123 = Close File(refnum=w153, error in=w152) -> ()  [unwired: 2 out]
                      }
                      frame True {
                      }
                    }
                    n124 = case shown="True" "Record MAP data?" {
                      frame False {
                      }
                      frame True {
                        n125 = while {
                          stop <- w167 stop-if-true
                          n126 = local read "File Name:"() -> (w162:string)
                          n127 = local read "Data Save Directory:"() -> (w166:path)
                          n128 = Concatenate Strings(w162, "_MAP") -> (w165:string)
                          n129 = call "DAQ Assistant15"("rate"="Sampling Rate (Hz)", "number of samples"="Number Samples", "device name"="ExternalADC") -> ("data"=w159:dynamicdata)  [unwired: 13 in, 3 out]
                          "NIBP Data (*scaled by 98 to convert from V to mmHg)" <- w159
                          n130 = local read "Mark #"() -> (w160:u32)
                          n131 = Merge Signals(w159, w160) -> (w161:dynamicdata)
                          n132 = Build Path(base path=w166, name or relative path=w165) -> (appended path=w164:path)
                          n133 = call "Write To Measurement File"("Signals"=w161, "Filename"=w164) -> ()  [unwired: 15 in, 3 out]
                          n134 = local read "Stop"() -> (w167:bool)
                        }
                      }
                    }
                    n135 = local read "Fixed # of Frames"() -> (w140:u32)
                    n136 = Initialize Array(nan, w140) -> (w138:dbl[])
                    n137 = while {
                      tunnel: w145 -> [w201]
                      tunnel: w144 -> [w200]
                      tunnel: w143 -> [_]
                      shift-right: [w168] -> _
                      shift-left: w138 -> [w169]
                      stop <- w175 stop-if-true
                      # "Only runs Real Time Fitting if \nReal Time Fitting box is checked \nand test function is off."
                      # "After everything is done, we have to\nbe nice and turn off them lasers and\nreset all the buttons."
                      n138 = for {
                        N: 1 -> [_]
                        tunnel: w200 -> [w248]
                        tunnel: w201 -> [w247]
                        tunnel: [w244] -> w175
                        tunnel: [w243] -> w198
                        tunnel: [w242] -> w179
                        tunnel: [w241] -> w178
                        tunnel: [w240] -> w177
                        # "The logic here may look funny but it works elegantly. No matter if you choose \"Use Both Lasers\", the AND output is always\nfalse the first time these two boxes run since Laser 1 Value is always false, and the default is to use flow laser 1.\nBUT, the trick is if you chose \"Use Both Laser\" This big for loop is gonna run twice, the second time it runs, \nthe laser 1 value is TRUE because it is set to TRUE by the second box when the big for loop ran the first time. Now, when\nthe output of AND is true, ISS laser no longer runs. Only flow laser two is turned on and we execute the for loop to the right."
                        # "These two boxes take care of the flow chart.\nIt turn on ISS laser first, then triggers it and turn it off.\nIf ISS data is ready, then we go on to flow lase."
                        # "This loop may seem useless but it acts as a block. \nThis block does all the data collection, plotting and writing the data\nto file"
                        n139 = stacked-sequence {
                          tunnel: [_ _ _ _ _ _ w271] -> w239
                          frame #0 {
                            # "DCS LASER OFF"
                            # "Turn relay off so that Optical switch is closed and LED indicator is OFF"
                            n140 = Build Array(FALSE, FALSE) -> (w251:bool[])
                            n141 = call "DAQ Assistant9"("data"=w251) -> ()  [unwired: 17 in, 2 out]
                            n142 = call "iBs.vi"("Laser On/Off"=FALSE, "VISA resource name"="Laser Input Name") -> ()
                          }
                          frame #1 {
                            # "ISS lasers ON"
                            n143 = Wait (ms)(milliseconds to wait=u32 100) -> ()  [unwired: 1 out]
                            n144 = Build Array(TRUE) -> (w255:bool[])
                            n145 = call "DAQ Assistant10"("data"=w255) -> ()  [unwired: 17 in, 2 out]
                          }
                          frame #2 {
                            n146 = stacked-sequence {
                              frame #0 {
                                # "ISS Data TRIGGER"
                                n147 = Build Array(TRUE) -> (w258:bool[])
                                n148 = call "DAQ Assistant12"("data"=w258) -> ()  [unwired: 17 in, 2 out]
                              }
                              frame #1 {
                                n149 = Wait (ms)(milliseconds to wait=u32 1000) -> ()  [unwired: 1 out]
                              }
                            }
                          }
                          frame #3 {
                            # "Make sure a second trigger isnt caught by turning trigger signal LOW"
                            n150 = Build Array(FALSE) -> (w260:bool[])
                            n151 = call "DAQ Assistant13"("data"=w260) -> ()  [unwired: 17 in, 2 out]
                          }
                          frame #4 {
                            # "Wait for AQ Active signal from ISS to go LOW"
                            n152 = while {
                              stop <- w262 continue-if-true
                              # "Loop until Dig Input signal is false"
                              n153 = Wait Until Next ms Multiple(millisecond multiple=u32 100 ("milliseconds to wait")) -> ()  [unwired: 1 out]
                              n154 = call "DAQ Assistant7"() -> ("data"=w263:bool[])  [unwired: 17 in, 2 out]
                              n155 = And Array Elements(Boolean array=w263) -> (logical AND=w262:bool)
                            }
                          }
                          frame #5 {
                            # "ISS lasers OFF"
                            # "Wait 500ms and then move on"
                            n156 = while {
                              stop <- TRUE stop-if-true
                              n157 = Wait (ms)(milliseconds to wait=500) -> ()  [unwired: 1 out]
                            }
                            n158 = Build Array(FALSE) -> (w265:bool[])
                            n159 = call "DAQ Assistant"("data"=w265) -> ()  [unwired: 17 in, 2 out]
                          }
                          frame #6 {
                            # "DCS LASER ON"
                            # "Turn relay ON so that Optical switch is open and LED indicator is ON"
                            n160 = Build Array(TRUE, TRUE) -> (w272:bool[])
                            n161 = local read "Laser Input Name"() -> (w269:refnum<visa-resource-name>)
                            n162 = call "DAQ Assistant11"("data"=w272) -> ()  [unwired: 17 in, 2 out]
                            n163 = call "iBs.vi"("Laser On/Off"=TRUE, "VISA resource name"=w269) -> ()
                            n164 = while {
                              tunnel: [w275] -> w271
                              stop <- w275 stop-if-true
                              w275 = TRUE
                              n165 = Wait (ms)(milliseconds to wait=200) -> ()  [unwired: 1 out]
                            }
                          }
                        }
                        n166 = case shown="\"8 Detectors\", Default" w247 {
                          selector: w247 -> [w610 w611]
                          tunnel: [w610 w611] -> w245
                          tunnel: w239 -> [_ _]
                          frame "4 Detectors" {
                            n167 = dll-call lib="C:/Users/BUCKLEY-ADMIN/Desktop/DCScode_simulISS_MAP/flex05-4chPascal.dll" fn="USBStart" label="StartCH4"() -> ()  [unwired: 4 in, 2 out]
                          }
                          frame "8 Detectors", Default {
                            n168 = dll-call lib="C:/Users/BUCKLEY-ADMIN/Desktop/DCScode_simulISS_MAP/flex05oem8chauto100nsPASCAL_win7.dll" fn="USBStart" label="StartCH8"() -> ()  [unwired: 4 in, 2 out]
                          }
                        }
                        n169 = for {
                          N: 1 -> [_]
                          tunnel: w248 -> [w297]
                          tunnel: [w281] -> w244
                          tunnel: w245 -> [w286]
                          tunnel: [w289] -> w243
                          tunnel: "MARK\nMark" -> [w288]
                          tunnel: [w287] -> w242
                          tunnel: [w279] -> w241
                          tunnel: [w285] -> w240
                          w298 = FALSE
                          w307 = u8 2
                          # "Only saves data if\ntest function is off."
                          # "If Fixed # Frames check box is selected,\ncode will run for # of frames specified on \nfront panel and then call Stop button"
                          # "This for loop here acts as a block as well. It takes the relative \nflow data from UpdateData.vi and plot the data on the graph.\nWhen \"Baseline\" is selected,  the data point goes to 1. When\n\"Mark\" is selected, a point at positive infinity is plotted and a\nvertical line joining the point and the x axis if displayed."
                          n170 = while {
                            tunnel: [w478] -> w306
                            tunnel: [w479] -> w305
                            tunnel: [w452] -> w304
                            tunnel: [w450] -> w281
                            tunnel: [w480] -> w303
                            tunnel: w297 -> [w482]
                            tunnel: w286 -> [w453]
                            stop <- w485 stop-if-true
                            n171 = Not(x="D3") -> (.not. x?=w467:bool)
                            n172 = Not(x="D4") -> (.not. x?=w466:bool)
                            n173 = Not(x="D8") -> (.not. x?=w462:bool)
                            n174 = Not(x="D5") -> (.not. x?=w465:bool)
                            n175 = Not(x="D1") -> (.not. x?=w469:bool)
                            n176 = Not(x="D6") -> (.not. x?=w464:bool)
                            n177 = Not(x="D2") -> (.not. x?=w454:bool)
                            n178 = Not(x="D7") -> (.not. x?=w463:bool)
                            n179 = case shown="True" "Stop" {
                              selector: "Stop" -> [w524 w531]
                              tunnel: [w524 w528] -> w450
                              frame False {
                              }
                              frame True {
                                # "Turn relay off so that Optical switch is closed and LED indicator is OFF"
                                n180 = call "Prompt User for Input"("Enable"=w531) -> ("Yes"=w528:bool)  [unwired: 17 in, 1 out]
                                n181 = local read "Laser Input Name"() -> (w525:refnum<visa-resource-name>)
                                n182 = Not(x=w528) -> (.not. x?=w527:bool)
                                n183 = Build Array(w527, FALSE) -> (w530:bool[])
                                n184 = call "DAQ Assistant2"("data"=w530) -> ()  [unwired: 17 in, 2 out]
                                n185 = call "iBs.vi"("Laser On/Off"=FALSE, "VISA resource name"=w525) -> ()
                              }
                            }
                            n186 = case shown="True" "Clear plots" {
                              frame False {
                              }
                              frame True {
                                n187 = invoke on="g2" class="XYGraph (strict)" method="Reinit To Default"() -> ()  [unwired: 3 in, 3 out]
                                n188 = property on="Tau" class="WFChart (strict)"("History Data"=cluster{"tmp":dbl, dbl}[] []) -> ()  [unwired: 2 in, 2 out]
                              }
                            }
                            n189 = case shown="True" w467 {
                              selector: w467 -> [w574 w575]
                              frame False {
                                n190 = property on="g2" class="XYGraph (strict)"("Active Plot"=u32 2) -> (error out=w572:errorcluster)  [unwired: 2 in, 1 out]
                                n191 = property on="g2" class="XYGraph (strict)"(error in=w572, "Plot.Visible?"=w574) -> ()  [unwired: 1 in, 2 out]
                              }
                              frame True {
                                n192 = property on="Tau 2" class="WFChart (strict)"("Active Plot"=u32 2) -> (error out=w577:errorcluster)  [unwired: 2 in, 1 out]
                                n193 = property on="Tau 2" class="WFChart (strict)"(error in=w577, "Plot.Visible?"=w575) -> ()  [unwired: 1 in, 2 out]
                                n194 = property on="g2" class="XYGraph (strict)"("Active Plot"=u32 2) -> (error out=w578:errorcluster)  [unwired: 2 in, 1 out]
                                n195 = property on="g2" class="XYGraph (strict)"(error in=w578, "Plot.Visible?"=w575) -> ()  [unwired: 1 in, 2 out]
                              }
                            }
                            n196 = case shown="True" w466 {
                              selector: w466 -> [w566 w567]
                              frame False {
                                n197 = property on="g2" class="XYGraph (strict)"("Active Plot"=u32 3) -> (error out=w564:errorcluster)  [unwired: 2 in, 1 out]
                                n198 = property on="g2" class="XYGraph (strict)"(error in=w564, "Plot.Visible?"=w566) -> ()  [unwired: 1 in, 2 out]
                              }
                              frame True {
                                n199 = property on="Tau 2" class="WFChart (strict)"("Active Plot"=u32 3) -> (error out=w568:errorcluster)  [unwired: 2 in, 1 out]
                                n200 = property on="Tau 2" class="WFChart (strict)"(error in=w568, "Plot.Visible?"=w567) -> ()  [unwired: 1 in, 2 out]
                                n201 = property on="g2" class="XYGraph (strict)"("Active Plot"=u32 3) -> (error out=w570:errorcluster)  [unwired: 2 in, 1 out]
                                n202 = property on="g2" class="XYGraph (strict)"(error in=w570, "Plot.Visible?"=w567) -> ()  [unwired: 1 in, 2 out]
                              }
                            }
                            n203 = case shown="True" w462 {
                              selector: w462 -> [w534 w535]
                              frame False {
                                n204 = property on="g2" class="XYGraph (strict)"("Active Plot"=u32 7) -> (error out=w532:errorcluster)  [unwired: 2 in, 1 out]
                                n205 = property on="g2" class="XYGraph (strict)"(error in=w532, "Plot.Visible?"=w534) -> ()  [unwired: 1 in, 2 out]
                              }
                              frame True {
                                n206 = property on="Tau 2" class="WFChart (strict)"("Active Plot"=u32 7) -> (error out=w537:errorcluster)  [unwired: 2 in, 1 out]
                                n207 = property on="Tau 2" class="WFChart (strict)"(error in=w537, "Plot.Visible?"=w535) -> ()  [unwired: 1 in, 2 out]
                                n208 = property on="g2" class="XYGraph (strict)"("Active Plot"=u32 7) -> (error out=w538:errorcluster)  [unwired: 2 in, 1 out]
                                n209 = property on="g2" class="XYGraph (strict)"(error in=w538, "Plot.Visible?"=w535) -> ()  [unwired: 1 in, 2 out]
                              }
                            }
                            n210 = case shown="True" w465 {
                              selector: w465 -> [w558 w559]
                              frame False {
                                n211 = property on="g2" class="XYGraph (strict)"("Active Plot"=u32 4) -> (error out=w556:errorcluster)  [unwired: 2 in, 1 out]
                                n212 = property on="g2" class="XYGraph (strict)"(error in=w556, "Plot.Visible?"=w558) -> ()  [unwired: 1 in, 2 out]
                              }
                              frame True {
                                n213 = property on="Tau 2" class="WFChart (strict)"("Active Plot"=u32 4) -> (error out=w561:errorcluster)  [unwired: 2 in, 1 out]
                                n214 = property on="Tau 2" class="WFChart (strict)"(error in=w561, "Plot.Visible?"=w559) -> ()  [unwired: 1 in, 2 out]
                                n215 = property on="g2" class="XYGraph (strict)"("Active Plot"=u32 4) -> (error out=w562:errorcluster)  [unwired: 2 in, 1 out]
                                n216 = property on="g2" class="XYGraph (strict)"(error in=w562, "Plot.Visible?"=w559) -> ()  [unwired: 1 in, 2 out]
                              }
                            }
                            n217 = case shown="True" w469 {
                              selector: w469 -> [w591 w592]
                              frame False {
                                n218 = property on="g2" class="XYGraph (strict)"("Active Plot"=u32 0) -> (error out=w589:errorcluster)  [unwired: 2 in, 1 out]
                                n219 = property on="g2" class="XYGraph (strict)"(error in=w589, "Plot.Visible?"=w591) -> ()  [unwired: 1 in, 2 out]
                              }
                              frame True {
                                n220 = property on="Tau 2" class="WFChart (strict)"("Active Plot"=u32 0) -> (error out=w594:errorcluster)  [unwired: 2 in, 1 out]
                                n221 = property on="Tau 2" class="WFChart (strict)"(error in=w594, "Plot.Visible?"=w592) -> ()  [unwired: 1 in, 2 out]
                                n222 = property on="g2" class="XYGraph (strict)"("Active Plot"=u32 0) -> (error out=w595:errorcluster)  [unwired: 2 in, 1 out]
                                n223 = property on="g2" class="XYGraph (strict)"(error in=w595, "Plot.Visible?"=w592) -> ()  [unwired: 1 in, 2 out]
                              }
                            }
                            n224 = case shown="True" w464 {
                              selector: w464 -> [w550 w551]
                              frame False {
                                n225 = property on="g2" class="XYGraph (strict)"("Active Plot"=u32 5) -> (error out=w548:errorcluster)  [unwired: 2 in, 1 out]
                                n226 = property on="g2" class="XYGraph (strict)"(error in=w548, "Plot.Visible?"=w550) -> ()  [unwired: 1 in, 2 out]
                              }
                              frame True {
                                n227 = property on="Tau 2" class="WFChart (strict)"("Active Plot"=u32 5) -> (error out=w552:errorcluster)  [unwired: 2 in, 1 out]
                                n228 = property on="Tau 2" class="WFChart (strict)"(error in=w552, "Plot.Visible?"=w551) -> ()  [unwired: 1 in, 2 out]
                                n229 = property on="g2" class="XYGraph (strict)"("Active Plot"=u32 5) -> (error out=w554:errorcluster)  [unwired: 2 in, 1 out]
                                n230 = property on="g2" class="XYGraph (strict)"(error in=w554, "Plot.Visible?"=w551) -> ()  [unwired: 1 in, 2 out]
                              }
                            }
                            n231 = case shown="True" w454 {
                              selector: w454 -> [w582 w583]
                              frame False {
                                n232 = property on="g2" class="XYGraph (strict)"("Active Plot"=u32 1) -> (error out=w580:errorcluster)  [unwired: 2 in, 1 out]
                                n233 = property on="g2" class="XYGraph (strict)"(error in=w580, "Plot.Visible?"=w582) -> ()  [unwired: 1 in, 2 out]
                              }
                              frame True {
                                n234 = property on="Tau 2" class="WFChart (strict)"("Active Plot"=u32 1) -> (error out=w585:errorcluster)  [unwired: 2 in, 1 out]
                                n235 = property on="Tau 2" class="WFChart (strict)"(error in=w585, "Plot.Visible?"=w583) -> ()  [unwired: 1 in, 2 out]
                                n236 = property on="g2" class="XYGraph (strict)"("Active Plot"=u32 1) -> (error out=w586:errorcluster)  [unwired: 2 in, 1 out]
                                n237 = property on="g2" class="XYGraph (strict)"(error in=w586, "Plot.Visible?"=w583) -> ()  [unwired: 1 in, 2 out]
                              }
                            }
                            n238 = case shown="True" w463 {
                              selector: w463 -> [w542 w543]
                              frame False {
                                n239 = property on="g2" class="XYGraph (strict)"("Active Plot"=u32 6) -> (error out=w540:errorcluster)  [unwired: 2 in, 1 out]
                                n240 = property on="g2" class="XYGraph (strict)"(error in=w540, "Plot.Visible?"=w542) -> ()  [unwired: 1 in, 2 out]
                              }
                              frame True {
                                n241 = property on="Tau 2" class="WFChart (strict)"("Active Plot"=u32 6) -> (error out=w544:errorcluster)  [unwired: 2 in, 1 out]
                                n242 = property on="Tau 2" class="WFChart (strict)"(error in=w544, "Plot.Visible?"=w543) -> ()  [unwired: 1 in, 2 out]
                                n243 = property on="g2" class="XYGraph (strict)"("Active Plot"=u32 6) -> (error out=w546:errorcluster)  [unwired: 2 in, 1 out]
                                n244 = property on="g2" class="XYGraph (strict)"(error in=w546, "Plot.Visible?"=w543) -> ()  [unwired: 1 in, 2 out]
                              }
                            }
                            n245 = call "UpdateData.vi"("Duration Time (ms)"="Integration Time (ms)", "Detector Select"=w453, "Delay Time"=w482) -> ("Elapsed Time(s)"=w484:sgl, "Intensity Array"=w481:sgl[], "Tau Array"=w480:sgl[], "Intensity data"=w478:string, "g2 Display"=→"g2":cluster{"Delay Time":sgl[], sgl[]}[], "tau data"=w479:string, "g2 data"=w452:string)  [unwired: 2 in, 8 out]
                            n246 = Wait (ms)(milliseconds to wait="Update Time (ms)\nDO NOT CHANGE!") -> ()  [unwired: 1 out]
                            n247 = Multiply(x=sgl 1000.0, y=w484) -> (x*y=w488:sgl)
                            n248 = Index Array(array=w481, index #1=0, index #2=1, index #3=2, index #4=3, index #5=4, index #6=5, index #7=6, index #8=7) -> (element #1=w384:sgl, element #2=w383:sgl, element #3=w382:sgl, element #4=w381:sgl, element #5=w380:sgl, element #6=w379:sgl, element #7=w378:sgl, element #8=w377:sgl)
                            "Det 7" <- w378
                            "Det 6" <- w379
                            "Det 5" <- w380
                            "Det 4" <- w381
                            "Det 3" <- w382
                            "Det 2" <- w383
                            "Det 1" <- w384
                            "Det 8" <- w377
                            n249 = Subtract(x="Integration Time (ms)", y=w488) -> (x-y=w486:sgl)
                            "Time Left (ms)" <- w486
                            n250 = Greater Or Equal?(x=w384, y=sgl 2.0) -> (x >= y?=w446:bool)
                            n251 = Greater Or Equal?(x=w383, y=sgl 2.0) -> (x >= y?=w441:bool)
                            n252 = Greater Or Equal?(x=w382, y=sgl 2.0) -> (x >= y?=w436:bool)
                            n253 = Greater Or Equal?(x=w381, y=sgl 2.0) -> (x >= y?=w431:bool)
                            n254 = Greater?(x=w384, y=0.98) -> (0:w362:bool)
                            n255 = Greater?(x=w383, y=0.98) -> (0:w364:bool)
                            n256 = Greater?(x=w382, y=0.98) -> (0:w366:bool)
                            n257 = Greater?(x=w381, y=0.98) -> (0:w368:bool)
                            n258 = Less Or Equal?(x=w384, y=sgl 1000.0) -> (x <= y?=w447:bool)
                            n259 = Less Or Equal?(x=w383, y=sgl 1000.0) -> (x <= y?=w440:bool)
                            n260 = Less Or Equal?(x=w382, y=sgl 1000.0) -> (x <= y?=w435:bool)
                            n261 = Less Or Equal?(x=w381, y=sgl 1000.0) -> (x <= y?=w430:bool)
                            n262 = Less Or Equal?(x=w380, y=sgl 1000.0) -> (x <= y?=w425:bool)
                            n263 = Less Or Equal?(x=w379, y=sgl 1000.0) -> (x <= y?=w420:bool)
                            n264 = Less Or Equal?(x=w378, y=sgl 1000.0) -> (x <= y?=w415:bool)
                            n265 = Less Or Equal?(x=w377, y=sgl 1000.0) -> (x <= y?=w410:bool)
                            n266 = Less?(x=w384, y=1.005) -> (x < y?=w361:bool)
                            n267 = Less?(x=w383, y=1.005) -> (x < y?=w363:bool)
                            n268 = Less?(x=w382, y=1.005) -> (x < y?=w365:bool)
                            n269 = Less?(x=w381, y=1.005) -> (x < y?=w367:bool)
                            n270 = Less?(x=w380, y=1.005) -> (x < y?=w369:bool)
                            n271 = Less?(x=w379, y=1.005) -> (x < y?=w371:bool)
                            n272 = Less?(x=w378, y=1.005) -> (x < y?=w373:bool)
                            n273 = Less?(x=w377, y=1.005) -> (x < y?=w375:bool)
                            n274 = Greater Or Equal?(x=w380, y=sgl 2.0) -> (x >= y?=w426:bool)
                            n275 = Greater Or Equal?(x=w379, y=sgl 2.0) -> (x >= y?=w421:bool)
                            n276 = Greater Or Equal?(x=w378, y=sgl 2.0) -> (x >= y?=w416:bool)
                            n277 = Greater Or Equal?(x=w377, y=sgl 2.0) -> (x >= y?=w411:bool)
                            n278 = Greater?(x=w380, y=0.98) -> (0:w370:bool)
                            n279 = Greater?(x=w379, y=0.98) -> (0:w372:bool)
                            n280 = Greater?(x=w378, y=0.98) -> (0:w374:bool)
                            n281 = Greater?(x=w377, y=0.98) -> (0:w376:bool)
                            n282 = Build Array(w361, w362, w446, w447) -> (w448:bool[])
                            n283 = Build Array(w364, w363, w441, w440) -> (w439:bool[])
                            n284 = Build Array(w365, w366, w436, w435) -> (w434:bool[])
                            n285 = Build Array(w368, w367, w431, w430) -> (w429:bool[])
                            n286 = Build Array(w370, w369, w426, w425) -> (w424:bool[])
                            n287 = Build Array(w372, w371, w421, w420) -> (w419:bool[])
                            n288 = Build Array(w374, w373, w416, w415) -> (w414:bool[])
                            n289 = Build Array(w375, w376, w411, w410) -> (w409:bool[])
                            n290 = And Array Elements(Boolean array=w448) -> (logical AND=w408:bool)
                            n291 = And Array Elements(Boolean array=w439) -> (logical AND=w407:bool)
                            n292 = And Array Elements(Boolean array=w434) -> (logical AND=w406:bool)
                            n293 = And Array Elements(Boolean array=w429) -> (logical AND=w405:bool)
                            n294 = And Array Elements(Boolean array=w424) -> (logical AND=w404:bool)
                            n295 = And Array Elements(Boolean array=w419) -> (logical AND=w403:bool)
                            n296 = And Array Elements(Boolean array=w414) -> (logical AND=w402:bool)
                            n297 = And Array Elements(Boolean array=w409) -> (logical AND=w401:bool)
                            n298 = Less Or Equal To 0?(x=w486) -> (x <= 0?=w487:bool)
                            n299 = case shown="False" w408 {
                              frame False {
                                n300 = control-ref of="Det 1"() -> (w520:refnum<vi>)
                                n301 = property on="Property Node" class="Digital (strict)"(reference=w520, "DisabledEnum"=T4."Disabled and Grayed Out" ("Disabled")) -> ()  [unwired: 1 in, 2 out]
                              }
                              frame True {
                                n302 = control-ref of="Det 1"() -> (w522:refnum<vi>)
                                n303 = property on="Property Node" class="Digital (strict)"(reference=w522, "DisabledEnum"=T4."Enabled" ("Disabled")) -> ()  [unwired: 1 in, 2 out]
                              }
                            }
                            n304 = case shown="False" w407 {
                              frame False {
                                n305 = control-ref of="Det 2"() -> (w516:refnum<vi>)
                                n306 = property on="Property Node" class="Digital (strict)"(reference=w516, "DisabledEnum"=T4."Disabled and Grayed Out" ("Disabled")) -> ()  [unwired: 1 in, 2 out]
                              }
                              frame True {
                                n307 = control-ref of="Det 2"() -> (w518:refnum<vi>)
                                n308 = property on="Property Node" class="Digital (strict)"(reference=w518, "DisabledEnum"=T4."Enabled" ("Disabled")) -> ()  [unwired: 1 in, 2 out]
                              }
                            }
                            n309 = case shown="False" w406 {
                              frame False {
                                n310 = control-ref of="Det 3"() -> (w512:refnum<vi>)
                                n311 = property on="Property Node" class="Digital (strict)"(reference=w512, "DisabledEnum"=T4."Disabled and Grayed Out" ("Disabled")) -> ()  [unwired: 1 in, 2 out]
                              }
                              frame True {
                                n312 = control-ref of="Det 3"() -> (w514:refnum<vi>)
                                n313 = property on="Property Node" class="Digital (strict)"(reference=w514, "DisabledEnum"=T4."Enabled" ("Disabled")) -> ()  [unwired: 1 in, 2 out]
                              }
                            }
                            n314 = case shown="False" w405 {
                              frame False {
                                n315 = control-ref of="Det 4"() -> (w508:refnum<vi>)
                                n316 = property on="Property Node" class="Digital (strict)"(reference=w508, "DisabledEnum"=T4."Disabled and Grayed Out" ("Disabled")) -> ()  [unwired: 1 in, 2 out]
                              }
                              frame True {
                                n317 = control-ref of="Det 4"() -> (w510:refnum<vi>)
                                n318 = property on="Property Node" class="Digital (strict)"(reference=w510, "DisabledEnum"=T4."Enabled" ("Disabled")) -> ()  [unwired: 1 in, 2 out]
                              }
                            }
                            n319 = case shown="False" w404 {
                              frame False {
                                n320 = control-ref of="Det 5"() -> (w504:refnum<vi>)
                                n321 = property on="Property Node" class="Digital (strict)"(reference=w504, "DisabledEnum"=T4."Disabled and Grayed Out" ("Disabled")) -> ()  [unwired: 1 in, 2 out]
                              }
                              frame True {
                                n322 = control-ref of="Det 5"() -> (w506:refnum<vi>)
                                n323 = property on="Property Node" class="Digital (strict)"(reference=w506, "DisabledEnum"=T4."Enabled" ("Disabled")) -> ()  [unwired: 1 in, 2 out]
                              }
                            }
                            n324 = case shown="True" w403 {
                              frame False {
                                n325 = control-ref of="Det 6"() -> (w500:refnum<vi>)
                                n326 = property on="Property Node" class="Digital (strict)"(reference=w500, "DisabledEnum"=T4."Disabled and Grayed Out" ("Disabled")) -> ()  [unwired: 1 in, 2 out]
                              }
                              frame True {
                                n327 = control-ref of="Det 6"() -> (w502:refnum<vi>)
                                n328 = property on="Property Node" class="Digital (strict)"(reference=w502, "DisabledEnum"=T4."Enabled" ("Disabled")) -> ()  [unwired: 1 in, 2 out]
                              }
                            }
                            n329 = case shown="True" w402 {
                              frame False {
                                n330 = control-ref of="Det 7"() -> (w496:refnum<vi>)
                                n331 = property on="Property Node" class="Digital (strict)"(reference=w496, "DisabledEnum"=T4."Disabled and Grayed Out" ("Disabled")) -> ()  [unwired: 1 in, 2 out]
                              }
                              frame True {
                                n332 = control-ref of="Det 7"() -> (w498:refnum<vi>)
                                n333 = property on="Property Node" class="Digital (strict)"(reference=w498, "DisabledEnum"=T4."Enabled" ("Disabled")) -> ()  [unwired: 1 in, 2 out]
                              }
                            }
                            n334 = case shown="True" w401 {
                              frame False {
                                n335 = control-ref of="Det 8"() -> (w492:refnum<vi>)
                                n336 = property on="Property Node" class="Digital (strict)"(reference=w492, "DisabledEnum"=T4."Disabled and Grayed Out" ("Disabled")) -> ()  [unwired: 1 in, 2 out]
                              }
                              frame True {
                                n337 = control-ref of="Det 8"() -> (w494:refnum<vi>)
                                n338 = property on="Property Node" class="Digital (strict)"(reference=w494, "DisabledEnum"=T4."Enabled" ("Disabled")) -> ()  [unwired: 1 in, 2 out]
                              }
                            }
                            n339 = Or(x=w450, y=w487) -> (x .or. y?=w485:bool)
                            n340 = case shown="True" w485 {
                              tunnel: w453 -> [w597 _]
                              frame True {
                                n341 = case shown="\"8 Detectors\", Default" w597 {
                                frame "4 Detectors" {
                                n342 = dll-call lib="C:/Users/BUCKLEY-ADMIN/Desktop/DCScode_simulISS_MAP/flex05-4chPascal.dll" fn="USBStop" label="StopCH4"() -> ()  [unwired: 4 in, 2 out]
                                }
                                frame "8 Detectors", Default {
                                n343 = dll-call lib="C:/Users/BUCKLEY-ADMIN/Desktop/DCScode_simulISS_MAP/flex05oem8chauto100nsPASCAL_win7.dll" fn="USBStop" label="StopCH8"() -> ()  [unwired: 4 in, 2 out]
                                }
                                }
                              }
                              frame False {
                              }
                            }
                          }
                          n344 = Current VI's Menubar() -> (w300:refnum<k9>)
                          n345 = local read "Trial #"() -> (w293:u32)
                          n346 = property on="QUIT" class="Bool"("Disabled"=w307) -> ()  [unwired: 2 in, 2 out]
                          n347 = Set Menu Item Info(7:"File", 9:w298, 11:w300) -> (3:w299:refnum<k9>)  [unwired: 4 in, 1 out]
                          n348 = Increment(x=w293) -> (x+1=w292:u32)
                          n349 = property on="Sequence Scan" class="Bool"("Disabled"=w307) -> ()  [unwired: 2 in, 2 out]
                          n350 = property on="Update Time (ms)\nDO NOT CHANGE!" class="DigNum (strict)"("Disabled"=w307) -> ()  [unwired: 2 in, 2 out]
                          n351 = property on="Integration Time (ms)" class="DigNum (strict)"("Disabled"=w307) -> ()  [unwired: 2 in, 2 out]
                          n352 = property on="Detector Select" class="RadioBtnsControl (strict)"("Disabled"=w307) -> ()  [unwired: 2 in, 2 out]
                          n353 = property on="Initialize Correlator" class="Bool"("Disabled"=w307) -> ()  [unwired: 2 in, 2 out]
                          n354 = local write "Trial #"(w292) -> ()
                          n355 = Set Menu Item Info(7:"Options", 9:w298, 11:w299) -> ()  [unwired: 4 in, 2 out]
                          n356 = case shown="\"Det 2\"" "Detector Used" {
                            tunnel: [1 2 3 4 5 6 7 8] -> w295
                            frame "Det 1", Default {
                            }
                            frame "Det 2" {
                            }
                            frame "Det 3" {
                            }
                            frame "Det 4" {
                            }
                            frame "Det 5" {
                            }
                            frame "Det 6" {
                            }
                            frame "Det 7" {
                            }
                            frame "Det 8" {
                            }
                          }
                          n357 = for {
                            N: 1 -> [_]
                            tunnel: w303 -> [w349]
                            tunnel: [w352] -> w296
                            tunnel: w295 -> [w351]
                            tunnel: w288 -> [w342]
                            n358 = case shown="True" w342 {
                              tunnel: [u32 0 w358] -> w352
                              frame False {
                              }
                              frame True {
                                n359 = local write "Trial #"(u32 0) -> ()
                                n360 = local read "Mark #"() -> (w360:u32)
                                n361 = Increment(x=w360) -> (x+1=w358:u32)
                                n362 = local write "Mark #"(w358) -> ()
                              }
                            }
                            n363 = Index Array(array=w349, index=w351) -> (element=w350:sgl)
                            n364 = Boolean To (0,1)(Boolean="Baseline") -> (0, 1=w354:i16)
                            n365 = case shown="False" w342 {
                              tunnel: [0.0 w356] -> w346
                              tunnel: inf -> [_ w356]
                              frame False {
                              }
                              frame True {
                              }
                            }
                            n366 = feedback #1() -> (w347:sgl)  [unwired: 1 in]
                            n367 = formula code="if(Tau==0) Tau=Tau+0.001;\nif(T==1) baselineflow=Tau;\n\ntmp=baselineflow/Tau;"("Tau"=w350, "T"=w354, "baselineflow"=w347) -> ("tmp"=w344:dbl, "baselineflow"=w348:sgl)
                            n368 = feedback-in #1(w348) -> ()
                            n369 = Bundle("tmp"=w344, w346) -> (→"Tau":cluster{"tmp":dbl, dbl})  [unwired: 1 in]
                          }
                          n370 = case shown="\"8 Detectors\", Default" w286 {
                            tunnel: w296 -> [w605 w609]
                            tunnel: [w606 w608] -> w313
                            tunnel: [4 8] -> w285
                            frame "4 Detectors" {
                              n371 = Build Array(w605, w605, w605, w605, w605) -> (w606:u32[])
                            }
                            frame "8 Detectors", Default {
                              n372 = Build Array(w609, w609, w609, w609, w609, w609, w609, w609, w609) -> (w608:u32[])
                            }
                          }
                          n373 = case shown="\"8 Detectors\", Default" w286 {
                            tunnel: ["%Duration\tID1\t\tID2\t\tID3\t\tID4\n" "%Duration\tID1\t\tID2\t\tID3\t\tID4\t\tID5\t\tID6\t\tID7\t\tID8\n"] -> w310
                            tunnel: ["%Tau\t\tTau1\t\tTau2\t\tTau3\t\tTau4\n" "%Tau\t\tTau1\t\tTau2\t\tTau3\t\tTau4\t\tTau5\t\tTau6\t\tTau7\t\tTau8\n"] -> w309
                            tunnel: ["%Delaytime\tD1\t\tD2\t\tD3\t\tD4\n" "%Delaytime\tD1\t\tD2\t\tD3\t\tD4\t\tD5\t\tD6\t\tD7\t\tD8\n"] -> w308
                            frame "4 Detectors" {
                            }
                            frame "8 Detectors", Default {
                            }
                          }
                          n374 = property on="Frame #" class="DigNum (strict)"() -> ("Value"=w279:u32)  [unwired: 2 in, 2 out]
                          n375 = case shown="True" "Fixed Time" {
                            tunnel: w279 -> [_ w333]
                            tunnel: [_ w330] -> w278
                            frame False {
                            }
                            frame True {
                              n376 = Increment(x="Fixed # of Frames") -> (x+1=w332:u32)
                              n377 = Less Or Equal?(x=w332, y=w333) -> (x <= y?=w330:bool)
                            }
                          }
                          n378 = Increment(x=w279) -> (x+1=w280:u32)
                          n379 = Number To Decimal String(number=w279) -> (decimal integer string=w314:string)  [unwired: 1 in]
                          n380 = Get Date/Time In Seconds() -> (seconds since 1Jan1904=w323:timestamp)
                          n381 = local write "Frame #"(w280) -> ()
                          n382 = Array To Spreadsheet String(array=w313, 3:"%d") -> (spreadsheet string=w311:string)  [unwired: 1 in]
                          n383 = Format Date/Time String(seconds (now)=w323) -> (date/time string=w320:string)  [unwired: 2 in]
                          "Computer Time" <- w320
                          n384 = Concatenate Strings("File Name:", "_flow_", w314, ".dat") -> (w283:string)
                          n385 = Concatenate Strings("%", w320, "\r\n", w310, w306, w309, "%\t\t", w305, w308, w304, w311) -> (w291:string)
                          n386 = Build Path(base path="Data Save Directory:", name or relative path=w283) -> (appended path=w290:path)
                          n387 = local read "Test"() -> (w277:bool)
                          n388 = case shown="False" w277 {
                            tunnel: w291 -> [w327 _]
                            tunnel: w290 -> [w326 _]
                            tunnel: [w325 _] -> w289
                            tunnel: [w324 _] -> w287
                            frame False {
                              n389 = Write to Text File(file (use dialog)=w326, text=w327) -> (refnum out=w328:refnum<file>, error out=w329:errorcluster)  [unwired: 2 in, 1 out]
                              n390 = Close File(refnum=w328, error in=w329) -> (path=w325:path, error out=w324:errorcluster)
                            }
                            frame True {
                            }
                          }
                          n391 = local write "Stop"(w278) -> ()
                        }
                      }
                      n392 = Index Array(array="Visible Averages", index=3) -> (element=w193:bool)
                      n393 = Index Array(array="Visible Averages", index=1) -> (element=w194:bool)
                      n394 = Index Array(array="Visible Averages", index=0) -> (element=w187:bool)
                      n395 = Index Array(array="Visible Averages", index=2) -> (element=w188:bool)
                      n396 = property on="Tau 2" class="WFChart (strict)"("Active Plot"=u32 11) -> (error out=w191:errorcluster)  [unwired: 2 in, 1 out]
                      n397 = property on="Tau 2" class="WFChart (strict)"("Active Plot"=u32 9) -> (error out=w196:errorcluster)  [unwired: 2 in, 1 out]
                      n398 = property on="Tau 2" class="WFChart (strict)"("Active Plot"=u32 8) -> (error out=w185:errorcluster)  [unwired: 2 in, 1 out]
                      n399 = property on="Tau 2" class="WFChart (strict)"("Active Plot"=u32 10) -> (error out=w190:errorcluster)  [unwired: 2 in, 1 out]
                      n400 = property on="Tau 2" class="WFChart (strict)"(error in=w191, "Plot.Visible?"=w193) -> ()  [unwired: 1 in, 2 out]
                      n401 = property on="Tau 2" class="WFChart (strict)"(error in=w196, "Plot.Visible?"=w194) -> ()  [unwired: 1 in, 2 out]
                      n402 = property on="Tau 2" class="WFChart (strict)"(error in=w185, "Plot.Visible?"=w187) -> ()  [unwired: 1 in, 2 out]
                      n403 = property on="Tau 2" class="WFChart (strict)"(error in=w190, "Plot.Visible?"=w188) -> ()  [unwired: 1 in, 2 out]
                      n404 = for {
                        N: 1 -> [_]
                        tunnel: w198 -> [_]
                        # "Turn relay off so that Optical switch is closed and LED indicator is OFF"
                        n405 = Build Array(FALSE, FALSE) -> (w234:bool[])
                        n406 = local read "Laser Input Name"() -> (w231:refnum<visa-resource-name>)
                        n407 = local write "Stop"(FALSE) -> ()
                        n408 = call "DAQ Assistant8"("data"=w234) -> ()  [unwired: 17 in, 2 out]
                        n409 = call "iBs.vi"("Laser On/Off"=FALSE, "VISA resource name"=w231) -> ()
                        n410 = Wait (ms)(milliseconds to wait="Delay between frames(ms)") -> ()  [unwired: 1 out]
                      }
                      n411 = Unbundle By Name(w179) -> ("status"=w197:bool)
                      n412 = local read "Test"() -> (w174:bool)
                      n413 = Not(x=w174) -> (.not. x?=w171:bool)
                      n414 = Not(x=w197) -> (.not. x?=w173:bool)
                      n415 = And(x="Real Time Fitting?", y=w171) -> (x .and. y?=w170:bool)
                      n416 = case shown="True" w170 {
                        tunnel: w173 -> [_ w207]
                        tunnel: w178 -> [_ w206]
                        tunnel: w177 -> [_ w205]
                        tunnel: w169 -> [w202 w204]
                        tunnel: [w202 w203] -> w168
                        frame False {
                        }
                        frame True {
                          n417 = case shown="True" w207 {
                            tunnel: w206 -> [_ w226]
                            tunnel: w205 -> [_ w222]
                            tunnel: w204 -> [w208 w220]
                            tunnel: [w208 w209] -> w203
                            frame False {
                            }
                            frame True {
                              # "Initialize Array of NaNs with size of \"fixed number of frames, \nand run this array into the case structure by putting it \nthrough a shift register with each loop it will replace one of \nthe NaNs by the flow data of the detector used. Then this data\nis averaged and COV is calculated."
                              n418 = property on="Data Save Directory:" class="Path"() -> ("Value"=w229:path)  [unwired: 2 in, 2 out]
                              n419 = property on="File Name:" class="Str"() -> ("Value"=w230:string)  [unwired: 2 in, 2 out]
                              n420 = call "GetFilePath.vi"("path"=w229, "file name"=w230, "frame number"=w226) -> ("final path C"=w221:string)  [unwired: 10 in, 2 out]
                              n421 = property on="Avg" class="Arr (strict)"() -> ("Value"=w227:bool[][])  [unwired: 2 in, 2 out]
                              n422 = local read "Detector Used"() -> (w219:T2)
                              n423 = call "DCSAnalysis.vi"("# Detectors"=w222, "File path"=w221, "Frame #"=w226, "rho"="rho", "other settings"="Other Settings", "avgBool"=w227, "var values"="Initial Guess") -> ("Flow in each detector"=w218:dbl[], "Tau"=→"Tau 2":T3)  [unwired: 18 in, 1 out]
                              "Flow in each detector" <- w218
                              n424 = Index Array(array=w218, index=w219) -> (element=w217:dbl)
                              n425 = local read "Trial #"() -> (w216:u32)
                              n426 = Decrement(x=w216) -> (x-1=w215:u32)
                              n427 = Replace Array Subset(array=w220, new element=w217, index=w215) -> (w209:dbl[])
                              n428 = call <vilib>:"Std Deviation and Variance.vi"("X"=w209) -> ("mean"=w213:dbl, "standard deviation"=w214:dbl)  [unwired: 1 in, 1 out]
                              "mean" <- w213
                              n429 = Divide(x=w214, y=w213) -> (x/y=w212:dbl)
                              n430 = Multiply(x=w212, y=100.0) -> (x*y=→"COV":dbl)
                            }
                          }
                        }
                      }
                    }
                  }
                  frame True {
                    n431 = invoke on="Sequence Scan" class="Bool" method="Reinit To Default"() -> ()  [unwired: 3 in, 3 out]
                    n432 = call "Display Message to User5"() -> ()  [unwired: 10 in, 2 out]
                  }
                }
              }
            }
            "Frame #" <- u32 0
            "Mark #" <- u32 0
            "Trial #" <- u32 0
          }
          event "QUIT": Value Change {
            # "Reset correlator before quitting"
            n433 = event-data() -> ()  [unwired: 1 in, 6 out]
            n434 = case shown="\"8 Detectors\", Default" w617 {
              frame "4 Detectors" {
                n435 = dll-call lib="C:/Users/BUCKLEY-ADMIN/Desktop/DCScode_simulISS_MAP/flex05-4chPascal.dll" fn="USBInitialize" label="InitCH4"() -> (error out=w619:errorcluster)  [unwired: 4 in, 1 out]
                n436 = dll-call lib="C:/Users/BUCKLEY-ADMIN/Desktop/DCScode_simulISS_MAP/flex05-4chPascal.dll" fn="USBFree" label="FreeCH4"(error in=w619) -> ()  [unwired: 3 in, 2 out]
              }
              frame "8 Detectors", Default {
                n437 = dll-call lib="C:/Users/BUCKLEY-ADMIN/Desktop/DCScode_simulISS_MAP/flex05oem8chauto100nsPASCAL_win7.dll" fn="USBInitialize" label="InitCH8"() -> (error out=w620:errorcluster)  [unwired: 4 in, 1 out]
                n438 = dll-call lib="C:/Users/BUCKLEY-ADMIN/Desktop/DCScode_simulISS_MAP/flex05oem8chauto100nsPASCAL_win7.dll" fn="USBFree" label="FreeCH8"(error in=w620) -> ()  [unwired: 3 in, 2 out]
              }
            }
            n439 = local write "Status"("Quit") -> ()
            n440 = local write "Status"("Quit") -> ()
          }
          event Timeout {
            w625 = TRUE
            w624 = u8 0
            # "This case structure turns on\n      and off the ISS Lasers"
            # "This case structure ensures that when the\noptical switch is turned on, the relay tells \nthe laser to power on."
            # "The system sits here and wait for some buttons to be pressed. And the status is always \"waiting\". Once some button is pressed, this value driven event\nstructure goes to the appropriate frame."
            n441 = event-data() -> ()  [unwired: 1 in, 3 out]
            n442 = local write "Status"("Waiting") -> ()
            n443 = property on="MARK\nMark" class="Bool"("DisabledEnum"=w624) -> ()  [unwired: 2 in, 2 out]
            n444 = property on="QUIT" class="Bool"("Disabled"=w624) -> ()  [unwired: 2 in, 2 out]
            n445 = property on="Sequence Scan" class="Bool"("Disabled"=w624) -> ()  [unwired: 2 in, 2 out]
            n446 = property on="Initialize Correlator" class="Bool"("Disabled"=w624) -> ()  [unwired: 2 in, 2 out]
            n447 = property on="Update Time (ms)\nDO NOT CHANGE!" class="DigNum (strict)"("Disabled"=w624) -> ()  [unwired: 2 in, 2 out]
            n448 = property on="Integration Time (ms)" class="DigNum (strict)"("Disabled"=w624) -> ()  [unwired: 2 in, 2 out]
            n449 = property on="Detector Select" class="RadioBtnsControl (strict)"("Disabled"=w624) -> ()  [unwired: 2 in, 2 out]
            n450 = case shown="True" "Optical Switch OPEN" {
              frame False {
                # "Send 2 signals, one for LED indicator, one for switch"
                n451 = Build Array(FALSE, FALSE) -> (w638:bool[])
                n452 = local read "Laser Input Name"() -> (w636:refnum<visa-resource-name>)
                n453 = call "DAQ Assistant3"("data"=w638) -> ()  [unwired: 17 in, 2 out]
                n454 = call "iBs.vi"("Laser On/Off"=FALSE, "VISA resource name"=w636) -> ()
              }
              frame True {
                n455 = Build Array(TRUE, TRUE) -> (w643:bool[])
                n456 = local read "Laser Input Name"() -> (w641:refnum<visa-resource-name>)
                n457 = call "DAQ Assistant4"("data"=w643) -> ()  [unwired: 17 in, 2 out]
                n458 = call "iBs.vi"("Laser On/Off"=TRUE, "VISA resource name"=w641) -> ()
              }
            }
            n459 = Current VI's Menubar() -> (w627:refnum<k9>)
            n460 = case shown="True" "ISS Lasers ON" {
              frame False {
                n461 = Build Array(FALSE) -> (w632:bool[])
                n462 = call "DAQ Assistant5"("data"=w632) -> ()  [unwired: 17 in, 2 out]
              }
              frame True {
                n463 = Build Array(TRUE) -> (w634:bool[])
                n464 = call "DAQ Assistant6"("data"=w634) -> ()  [unwired: 17 in, 2 out]
              }
            }
            n465 = Set Menu Item Info(7:"File", 9:w625, 11:w627) -> (3:w626:refnum<k9>)  [unwired: 4 in, 1 out]
            n466 = Set Menu Item Info(7:"Options", 9:w625, 11:w626) -> ()  [unwired: 4 in, 2 out]
            n467 = Get Date/Time In Seconds() -> (seconds since 1Jan1904=w630:timestamp)
            n468 = Format Date/Time String(seconds (now)=w630) -> (date/time string=w631:string)  [unwired: 2 in]
            n469 = local write "Computer Time"(w631) -> ()
          }
        }
      }
    }
  }
  n470 = local read "Laser Input Name"() -> (w1:refnum<visa-resource-name>)
  n471 = call "iBs.vi"("Laser On/Off"=FALSE, "VISA resource name"=w1) -> ()
